vi "globals.vi"() -> ()   [LabVIEW 2011]
uses:
  relaySpec.ctl
  DA_Spec.ctl
  AD_Spec.ctl
panel:
  in  "Global Variables":enum32{"General", "Card Slots", "Functions"}(tab)=enum."Functions"
  out "GPIB Address":string="23"
  out "Log File Path":path
  out "Byte Stream File Refnum":refnum<file>
  out "Log String":string="00:00 Begin sequence\r\n00:01 R_H2:API_Iterations(\"1\"),API_Seq_Num(\"1/30\"),Active,Flow1(720),Remote\r\n00:01 H_Heater:API_Iterations(\"1\"),API_Repetitions(\"1\"),API_Seq_Num(\"2/30\"),Remote,Spinner\r\n00:06 A_Change_Temp_Setpoint:API_Description(\"100 C\"),API_ID(\"11\"),API_Iterations(\"1\"),API_Mode(\"Instantaneous\"),API_Seq_Num(\"3/30\"),API_Start,Elapsed Time \\(s\\)(\"0\"),Prompt(\"Is temperature 100 C?\"),Setpoint \\(C\\)(\"100\")\r\n00:08 H_Heater:API_Iterations(\"1\"),API_Repetitions(\"1\"),API_Seq_Num(\"4/30\"),Heater,Remote,Spinner\r\n00:38 A_Change_Temp_Setpoint:API_Description(\"200 C\"),API_ID(\"14\"),API_Iterations(\"1\"),API_Mode(\"Instantaneous\"),API_Seq_Num(\"5/30\"),API_Start,Elapsed Time \\(s\\)(\"0\"),Prompt(\"Is temperature 200 C?\"),Setpoint \\(C\\)(\"200\")\r\n01:38 A_Change_Temp_Setpoint:API_Description(\"300 C\"),API_ID(\"1\"),API_Iterations(\"1\"),API_Mode(\"Instantaneous\"),API_Seq_Num(\"6/30\"),API_Start,Elapsed Time \\(s\\)(\"0\"),Prompt(\"Is temperature 300 C?\"),Setpoint \\(C\\)(\"300\")\r\n01:39 A_III_V_Layer_v23:API_Calculated_Time(\"60\"),API_ID(\"12\"),API_Iterations(\"1\"),API_Mode(\"Finite\"),API_Seq_Num(\"7/30\"),API_Start,Al_bubbler.Flow(\"0\"),Al_bubbler.Name(\"Al\"),As_gas.Active,As_gas.Flow(\"8\"),As_gas.Name(\"As gas\"),Comment(\"fill lines\"),Ga_bubbler.Calculated(\"0\"),Ga_bubbler.MFC1 flow(\"10\"),Ga_bubbler.MFC2 flow(\"0\"),Ga_bubbler.MFC3 flow(\"0\"),Ga_bubbler.Main.Active,Ga_bubbler.Main.Flow(\"10\"),Ga_bubbler.Main.Name(\"Ga\"),In_bubbler.Active,In_bubbler.Flow(\"10\"),In_bubbler.Name(\"In\"),P_bubbler.Flow(\"0\"),P_bubbler.Name(\"P liq\"),P_gas.Active,P_gas.Flow(\"10\"),P_gas.Name(\"P gas\"),Se_bubbler.Calculated(\"0\"),Se_bubbler.MFC1 flow(\"0\"),Se_bubbler.MFC2 flow(\"10\"),Se_bubbler.MFC3 flow(\"100\"),Se_bubbler.Main.Flow(\"0\"),Se_bubbler.Main.Name(\"Se\"),Zn_bubbler.Calculated(\"0\"),Zn_bubbler.MFC1 flow(\"0\"),Zn_bubbler.MFC2 flow(\"10\"),Zn_bubbler.MFC3 flow(\"100\"),Zn_bubbler.Main.Flow(\"0\"),Zn_bubbler.Main.Name(\"Zn\"),prep_time(\"0\")\r\n02:39 A_III_V_Layer_v23:API_Calculated_Time(\"0\"),API_ID(\"6\"),API_Iterations(\"1\"),API_Mode(\"Finite\"),API_Seq_Num(\"8/30\"),API_Start,Al_bubbler.Flow(\"0\"),Al_bubbler.Name(\"Al\"),As_gas.Active,As_gas.Flow(\"4\"),As_gas.Name(\"As gas\"),As_gas.Prep,As_gas.Run,Comment(\"AsH3\"),Ga_bubbler.Calculated(\"0\"),Ga_bubbler.MFC1 flow(\"0\"),Ga_bubbler.MFC2 flow(\"0\"),Ga_bubbler.MFC3 flow(\"0\"),Ga_bubbler.Main.Flow(\"0\"),Ga_bubbler.Main.Name(\"Ga\"),In_bubbler.Flow(\"0\"),In_bubbler.Name(\"In\"),P_bubbler.Flow(\"0\"),P_bubbler.Name(\"P liq\"),P_gas.Flow(\"0\"),P_gas.Name(\"P gas\"),Se_bubbler.Calculated(\"0\"),Se_bubbler.MFC1 flow(\"0\"),Se_bubbler.MFC2 flow(\"10\"),Se_bubbler.MFC3 flow(\"100\"),Se_bubbler.Main.Flow(\"0\"),Se_bubbler.Main.Name(\"Se\"),Zn_bubbler.Calculated(\"0\"),Zn_bubbler.MFC1 flow(\"0\"),Zn_bubbler.MFC2 flow(\"10\"),Zn_bubbler.MFC3 flow(\"100\"),Zn_bubbler.Main.Flow(\"0\"),Zn_bubbler.Main.Name(\"Zn\"),prep_time(\"0\")\r\n02:39 A_Change_Temp_Setpoint:API_Description(\"400 C\"),API_ID(\"13\"),API_Iterations(\"1\"),API_Mode(\"Instantaneous\"),API_Seq_Num(\"9/30\"),API_Start,Elapsed Time \\(s\\)(\"0\"),Prompt(\"Is temperature 400 C?\"),Setpoint \\(C\\)(\"400\")\r\n03:39 A_Change_Temp_Setpoint:API_Description(\"500 C\"),API_ID(\"15\"),API_Iterations(\"1\"),API_Mode(\"Instantaneous\"),API_Seq_Num(\"10/30\"),API_Start,Elapsed Time \\(s\\)(\"0\"),Prompt(\"Is temperature 500 C?\"),Setpoint \\(C\\)(\"500\")\r\n04:40 A_Change_Temp_Setpoint:API_Description(\"600 C\"),API_ID(\"3\"),API_Iterations(\"1\"),API_Mode(\"Instantaneous\"),API_Seq_Num(\"11/30\"),API_Start,Elapsed Time \\(s\\)(\"0\"),Prompt(\"Is temperature 600 C?\"),Setpoint \\(C\\)(\"600\")\r\n05:40 A_Change_Temp_Setpoint:API_Description(\"625 C\"),API_ID(\"20\"),API_Iterations(\"1\"),API_Mode(\"Instantaneous\"),API_Seq_Num(\"12/30\"),API_Start,Elapsed Time \\(s\\)(\"0\"),Prompt(\"Is temperature 625 C?\"),Setpoint \\(C\\)(\"625\")\r\n06:40 A_III_V_Layer_v23:API_Calculated_Time(\"0\"),API_ID(\"2\"),API_Iterations(\"1\"),API_Mode(\"Finite\"),API_Seq_Num(\"13/30\"),API_Start,Al_bubbler.Flow(\"0\"),Al_bubbler.Name(\"Al\"),As_gas.Active,As_gas.Flow(\"4\"),As_gas.Name(\"As gas\"),As_gas.Prep,As_gas.Run,Comment(\"prep\"),Ga_bubbler.Calculated(\"0\"),Ga_bubbler.Dilution,Ga_bubbler.MFC1 flow(\"10\"),Ga_bubbler.MFC2 flow(\"10\"),Ga_bubbler.MFC3 flow(\"100\"),Ga_bubbler.Main.Active,Ga_bubbler.Main.Flow(\"0.909091\"),Ga_bubbler.Main.Name(\"Ga\"),In_bubbler.Flow(\"0\"),In_bubbler.Name(\"In\"),P_bubbler.Flow(\"0\"),P_bubbler.Name(\"P liq\"),P_gas.Flow(\"0\"),P_gas.Name(\"P gas\"),Se_bubbler.Calculated(\"0\"),Se_bubbler.MFC1 flow(\"0\"),Se_bubbler.MFC2 flow(\"10\"),Se_bubbler.MFC3 flow(\"100\"),Se_bubbler.Main.Flow(\"0\"),Se_bubbler.Main.Name(\"Se\"),Zn_bubbler.Calculated(\"0\"),Zn_bubbler.MFC1 flow(\"0\"),Zn_bubbler.MFC2 flow(\"10\"),Zn_bubbler.MFC3 flow(\"100\"),Zn_bubbler.Main.Flow(\"0\"),Zn_bubbler.Main.Name(\"Zn\"),prep_time(\"0\")\r\n06:40 A_Change_Temp_Setpoint:API_Description(\"650 C\"),API_ID(\"16\"),API_Iterations(\"1\"),API_Mode(\"Instantaneous\"),API_Seq_Num(\"14/30\"),API_Start,Elapsed Time \\(s\\)(\"0\"),Prompt(\"Is temperature 650 C?\"),Setpoint \\(C\\)(\"650\")\r\n07:40 A_III_V_Layer_v23:API_Calculated_Time(\"300\"),API_ID(\"21\"),API_Iterations(\"1\"),API_Mode(\"Finite\"),API_Seq_Num(\"15/30\"),API_Start,Al_bubbler.Flow(\"0\"),Al_bubbler.Name(\"Al\"),As_gas.Active,As_gas.Flow(\"6\"),As_gas.Name(\"As gas\"),As_gas.Prep,As_gas.Run,Comment(\"GaAs buffer 1\"),Ga_bubbler.Calculated(\"0\"),Ga_bubbler.Dilution,Ga_bubbler.MFC1 flow(\"10\"),Ga_bubbler.MFC2 flow(\"10\"),Ga_bubbler.MFC3 flow(\"100\"),Ga_bubbler.Main.Active,Ga_bubbler.Main.Flow(\"0.909091\"),Ga_bubbler.Main.Name(\"Ga\"),Ga_bubbler.Main.Run,In_bubbler.Flow(\"0\"),In_bubbler.Name(\"In\"),P_bubbler.Flow(\"0\"),P_bubbler.Name(\"P liq\"),P_gas.Flow(\"0\"),P_gas.Name(\"P gas\"),Se_bubbler.Calculated(\"0\"),Se_bubbler.MFC1 flow(\"0\"),Se_bubbler.MFC2 flow(\"10\"),Se_bubbler.MFC3 flow(\"100\"),Se_bubbler.Main.Flow(\"0\"),Se_bubbler.Main.Name(\"Se\"),Zn_bubbler.Calculated(\"0\"),Zn_bubbler.MFC1 flow(\"0\"),Zn_bubbler.MFC2 flow(\"10\"),Zn_bubbler.MFC3 flow(\"100\"),Zn_bubbler.Main.Flow(\"0\"),Zn_bubbler.Main.Name(\"Zn\"),prep_time(\"60\")\r\n12:41 A_III_V_Layer_v23:API_Calculated_Time(\"124\"),API_ID(\"18\"),API_Iterations(\"1\"),API_Mode(\"Finite\"),API_Seq_Num(\"16/30\"),API_Start,Al_bubbler.Flow(\"0\"),Al_bubbler.Name(\"Al\"),As_gas.Active,As_gas.Flow(\"6\"),As_gas.Name(\"As gas\"),As_gas.Prep,As_gas.Run,Comment(\"GaAs buffer2\"),Ga_bubbler.Calculated(\"0\"),Ga_bubbler.Dilution,Ga_bubbler.MFC1 flow(\"10\"),Ga_bubbler.MFC2 flow(\"10\"),Ga_bubbler.MFC3 flow(\"100\"),Ga_bubbler.Main.Active,Ga_bubbler.Main.Flow(\"0.909091\"),Ga_bubbler.Main.Name(\"Ga\"),Ga_bubbler.Main.Run,In_bubbler.Active,In_bubbler.Flow(\"70\"),In_bubbler.Name(\"In\"),P_bubbler.Flow(\"0\"),P_bubbler.Name(\"P liq\"),P_gas.Active,P_gas.Flow(\"4\"),P_gas.Name(\"P gas\"),Se_bubbler.Calculated(\"0\"),Se_bubbler.MFC1 flow(\"0\"),Se_bubbler.MFC2 flow(\"10\"),Se_bubbler.MFC3 flow(\"100\"),Se_bubbler.Main.Flow(\"0\"),Se_bubbler.Main.Name(\"Se\"),Zn_bubbler.Calculated(\"0\"),Zn_bubbler.MFC1 flow(\"0\"),Zn_bubbler.MFC2 flow(\"10\"),Zn_bubbler.MFC3 flow(\"100\"),Zn_bubbler.Main.Flow(\"0\"),Zn_bubbler.Main.Name(\"Zn\"),prep_time(\"4\")\r\n14:46 A_III_V_Layer_v23:API_Calculated_Time(\"2\"),API_ID(\"8\"),API_Iterations(\"1\"),API_Mode(\"Finite\"),API_Seq_Num(\"17/30\"),API_Start,Al_bubbler.Flow(\"0\"),Al_bubbler.Name(\"Al\"),As_gas.Active,As_gas.Flow(\"4\"),As_gas.Name(\"As gas\"),As_gas.Prep,As_gas.Run,Comment(\"post buffer 2\"),Ga_bubbler.Calculated(\"0\"),Ga_bubbler.Dilution,Ga_bubbler.MFC1 flow(\"9.56\"),Ga_bubbler.MFC2 flow(\"10\"),Ga_bubbler.MFC3 flow(\"100\"),Ga_bubbler.Main.Active,Ga_bubbler.Main.Flow(\"0.872581\"),Ga_bubbler.Main.Name(\"Ga\"),In_bubbler.Active,In_bubbler.Flow(\"70\"),In_bubbler.Name(\"In\"),P_bubbler.Flow(\"0\"),P_bubbler.Name(\"P liq\"),P_gas.Active,P_gas.Flow(\"4\"),P_gas.Name(\"P gas\"),Se_bubbler.Calculated(\"0\"),Se_bubbler.MFC1 flow(\"0\"),Se_bubbler.MFC2 flow(\"10\"),Se_bubbler.MFC3 flow(\"100\"),Se_bubbler.Main.Flow(\"0\"),Se_bubbler.Main.Name(\"Se\"),Zn_bubbler.Calculated(\"0\"),Zn_bubbler.MFC1 flow(\"0\"),Zn_bubbler.MFC2 flow(\"10\"),Zn_bubbler.MFC3 flow(\"100\"),Zn_bubbler.Main.Flow(\"0\"),Zn_bubbler.Main.Name(\"Zn\"),prep_time(\"0\")\r\n14:48 A_III_V_Layer_v23:API_Calculated_Time(\"2\"),API_ID(\"9\"),API_Iterations(\"1\"),API_Mode(\"Finite\"),API_Seq_Num(\"18/30\"),API_Start,Al_bubbler.Flow(\"0\"),Al_bubbler.Name(\"Al\"),As_gas.Flow(\"0\"),As_gas.Name(\"As gas\"),Comment(\"nothing running\"),Ga_bubbler.Calculated(\"0\"),Ga_bubbler.Dilution,Ga_bubbler.MFC1 flow(\"9.56\"),Ga_bubbler.MFC2 flow(\"10\"),Ga_bubbler.MFC3 flow(\"100\"),Ga_bubbler.Main.Active,Ga_bubbler.Main.Flow(\"0.872581\"),Ga_bubbler.Main.Name(\"Ga\"),In_bubbler.Active,In_bubbler.Flow(\"70\"),In_bubbler.Name(\"In\"),P_bubbler.Flow(\"0\"),P_bubbler.Name(\"P liq\"),P_gas.Active,P_gas.Flow(\"4\"),P_gas.Name(\"P gas\"),Se_bubbler.Calculated(\"0\"),Se_bubbler.MFC1 flow(\"0\"),Se_bubbler.MFC2 flow(\"10\"),Se_bubbler.MFC3 flow(\"100\"),Se_bubbler.Main.Flow(\"0\"),Se_bubbler.Main.Name(\"Se\"),Zn_bubbler.Calculated(\"0\"),Zn_bubbler.MFC1 flow(\"0\"),Zn_bubbler.MFC2 flow(\"10\"),Zn_bubbler.MFC3 flow(\"100\"),Zn_bubbler.Main.Flow(\"0\"),Zn_bubbler.Main.Name(\"Zn\"),prep_time(\"0\")\r\n14:50 A_III_V_Layer_v23:API_Calculated_Time(\"3484\"),API_ID(\"19\"),API_Iterations(\"1\"),API_Mode(\"Finite\"),API_Seq_Num(\"19/30\"),API_Start,Al_bubbler.Flow(\"0\"),Al_bubbler.Name(\"Al\"),As_gas.Flow(\"0\"),As_gas.Name(\"As gas\"),Comment(\"GaInP\"),Ga_bubbler.Calculated(\"0\"),Ga_bubbler.Dilution,Ga_bubbler.MFC1 flow(\"9.56\"),Ga_bubbler.MFC2 flow(\"10\"),Ga_bubbler.MFC3 flow(\"100\"),Ga_bubbler.Main.Active,Ga_bubbler.Main.Flow(\"0.872581\"),Ga_bubbler.Main.Name(\"Ga\"),Ga_bubbler.Main.Run,In_bubbler.Active,In_bubbler.Flow(\"70\"),In_bubbler.Name(\"In\"),In_bubbler.Run,P_bubbler.Flow(\"0\"),P_bubbler.Name(\"P liq\"),P_gas.Active,P_gas.Flow(\"4\"),P_gas.Name(\"P gas\"),P_gas.Prep,P_gas.Run,Se_bubbler.Calculated(\"0\"),Se_bubbler.MFC1 flow(\"0\"),Se_bubbler.MFC2 flow(\"10\"),Se_bubbler.MFC3 flow(\"100\"),Se_bubbler.Main.Flow(\"0\"),Se_bubbler.Main.Name(\"Se\"),Zn_bubbler.Calculated(\"0\"),Zn_bubbler.MFC1 flow(\"0\"),Zn_bubbler.MFC2 flow(\"10\"),Zn_bubbler.MFC3 flow(\"100\"),Zn_bubbler.Main.Flow(\"0\"),Zn_bubbler.Main.Name(\"Zn\"),prep_time(\"4\")\r\n1:22:42 A_III_V_Layer_v23:API_Calculated_Time(\"120\"),API_ID(\"22\"),API_Iterations(\"1\"),API_Mode(\"Finite\"),API_Seq_Num(\"20/30\"),API_Start,Al_bubbler.Flow(\"0\"),Al_bubbler.Name(\"Al\"),As_gas.Active,As_gas.Flow(\"4\"),As_gas.Name(\"As gas\"),Comment(\"GaInP_end\"),Ga_bubbler.Calculated(\"0\"),Ga_bubbler.Dilution,Ga_bubbler.MFC1 flow(\"9.56\"),Ga_bubbler.MFC2 flow(\"10\"),Ga_bubbler.MFC3 flow(\"100\"),Ga_bubbler.Main.Active,Ga_bubbler.Main.Flow(\"0.872581\"),Ga_bubbler.Main.Name(\"Ga\"),Ga_bubbler.Main.Run,In_bubbler.Active,In_bubbler.Flow(\"70\"),In_bubbler.Name(\"In\"),In_bubbler.Run,P_bubbler.Flow(\"0\"),P_bubbler.Name(\"P liq\"),P_gas.Active,P_gas.Flow(\"4\"),P_gas.Name(\"P gas\"),P_gas.Prep,P_gas.Run,Se_bubbler.Calculated(\"0\"),Se_bubbler.MFC1 flow(\"0\"),Se_bubbler.MFC2 flow(\"10\"),Se_bubbler.MFC3 flow(\"100\"),Se_bubbler.Main.Flow(\"0\"),Se_bubbler.Main.Name(\"Se\"),Zn_bubbler.Calculated(\"0\"),Zn_bubbler.MFC1 flow(\"0\"),Zn_bubbler.MFC2 flow(\"10\"),Zn_bubbler.MFC3 flow(\"100\"),Zn_bubbler.Main.Flow(\"0\"),Zn_bubbler.Main.Name(\"Zn\"),prep_time(\"0\")\r\n1:24:42 A_III_V_Layer_v23:API_Calculated_Time(\"4\"),API_ID(\"23\"),API_Iterations(\"1\"),API_Mode(\"Finite\"),API_Seq_Num(\"21/30\"),API_Start,Al_bubbler.Flow(\"0\"),Al_bubbler.Name(\"Al\"),As_gas.Active,As_gas.Flow(\"4\"),As_gas.Name(\"As gas\"),Comment(\"post-GaInP\"),Ga_bubbler.Calculated(\"0\"),Ga_bubbler.Dilution,Ga_bubbler.MFC1 flow(\"10\"),Ga_bubbler.MFC2 flow(\"10\"),Ga_bubbler.MFC3 flow(\"100\"),Ga_bubbler.Main.Active,Ga_bubbler.Main.Flow(\"0.909091\"),Ga_bubbler.Main.Name(\"Ga\"),In_bubbler.Flow(\"0\"),In_bubbler.Name(\"In\"),P_bubbler.Flow(\"0\"),P_bubbler.Name(\"P liq\"),P_gas.Active,P_gas.Flow(\"4\"),P_gas.Name(\"P gas\"),P_gas.Prep,P_gas.Run,Se_bubbler.Calculated(\"0\"),Se_bubbler.MFC1 flow(\"0\"),Se_bubbler.MFC2 flow(\"10\"),Se_bubbler.MFC3 flow(\"100\"),Se_bubbler.Main.Flow(\"0\"),Se_bubbler.Main.Name(\"Se\"),Zn_bubbler.Calculated(\"0\"),Zn_bubbler.MFC1 flow(\"0\"),Zn_bubbler.MFC2 flow(\"10\"),Zn_bubbler.MFC3 flow(\"100\"),Zn_bubbler.Main.Flow(\"0\"),Zn_bubbler.Main.Name(\"Zn\"),prep_time(\"0\")\r\n1:24:46 A_III_V_Layer_v23:API_Calculated_Time(\"2\"),API_ID(\"4\"),API_Iterations(\"1\"),API_Mode(\"Finite\"),API_Seq_Num(\"22/30\"),API_Start,Al_bubbler.Flow(\"0\"),Al_bubbler.Name(\"Al\"),As_gas.Active,As_gas.Flow(\"4\"),As_gas.Name(\"As gas\"),Comment(\"no growth\"),Ga_bubbler.Calculated(\"0\"),Ga_bubbler.Dilution,Ga_bubbler.MFC1 flow(\"10\"),Ga_bubbler.MFC2 flow(\"10\"),Ga_bubbler.MFC3 flow(\"100\"),Ga_bubbler.Main.Active,Ga_bubbler.Main.Flow(\"0.909091\"),Ga_bubbler.Main.Name(\"Ga\"),In_bubbler.Flow(\"0\"),In_bubbler.Name(\"In\"),P_bubbler.Flow(\"0\"),P_bubbler.Name(\"P liq\"),P_gas.Flow(\"0\"),P_gas.Name(\"P gas\"),Se_bubbler.Calculated(\"0\"),Se_bubbler.MFC1 flow(\"0\"),Se_bubbler.MFC2 flow(\"10\"),Se_bubbler.MFC3 flow(\"100\"),Se_bubbler.Main.Flow(\"0\"),Se_bubbler.Main.Name(\"Se\"),Zn_bubbler.Calculated(\"0\"),Zn_bubbler.MFC1 flow(\"0\"),Zn_bubbler.MFC2 flow(\"10\"),Zn_bubbler.MFC3 flow(\"100\"),Zn_bubbler.Main.Flow(\"0\"),Zn_bubbler.Main.Name(\"Zn\"),prep_time(\"2\")\r\n1:24:49 A_III_V_Layer_v23:API_Calculated_Time(\"125\"),API_ID(\"5\"),API_Iterations(\"1\"),API_Mode(\"Finite\"),API_Seq_Num(\"23/30\"),API_Start,Al_bubbler.Flow(\"0\"),Al_bubbler.Name(\"Al\"),As_gas.Active,As_gas.Flow(\"4\"),As_gas.Name(\"As gas\"),As_gas.Prep,As_gas.Run,Comment(\"cap\"),Ga_bubbler.Calculated(\"0\"),Ga_bubbler.Dilution,Ga_bubbler.MFC1 flow(\"10\"),Ga_bubbler.MFC2 flow(\"10\"),Ga_bubbler.MFC3 flow(\"100\"),Ga_bubbler.Main.Active,Ga_bubbler.Main.Flow(\"0.909091\"),Ga_bubbler.Main.Name(\"Ga\"),Ga_bubbler.Main.Run,In_bubbler.Flow(\"0\"),In_bubbler.Name(\"In\"),P_bubbler.Flow(\"0\"),P_bubbler.Name(\"P liq\"),P_gas.Flow(\"0\"),P_gas.Name(\"P gas\"),Se_bubbler.Calculated(\"0\"),Se_bubbler.MFC1 flow(\"0\"),Se_bubbler.MFC2 flow(\"10\"),Se_bubbler.MFC3 flow(\"100\"),Se_bubbler.Main.Flow(\"0\"),Se_bubbler.Main.Name(\"Se\"),Zn_bubbler.Calculated(\"0\"),Zn_bubbler.MFC1 flow(\"0\"),Zn_bubbler.MFC2 flow(\"10\"),Zn_bubbler.MFC3 flow(\"100\"),Zn_bubbler.Main.Flow(\"0\"),Zn_bubbler.Main.Name(\"Zn\"),prep_time(\"5\")\r\n1:26:55 A_III_V_Layer_v23:API_Calculated_Time(\"0\"),API_ID(\"10\"),API_Iterations(\"1\"),API_Mode(\"Finite\"),API_Seq_Num(\"24/30\"),API_Start,Al_bubbler.Flow(\"0\"),Al_bubbler.Name(\"Al\"),As_gas.Active,As_gas.Flow(\"3\"),As_gas.Name(\"As gas\"),As_gas.Prep,As_gas.Run,Comment(\"post growth\"),Ga_bubbler.Calculated(\"0\"),Ga_bubbler.MFC1 flow(\"0\"),Ga_bubbler.MFC2 flow(\"0\"),Ga_bubbler.MFC3 flow(\"0\"),Ga_bubbler.Main.Flow(\"0\"),Ga_bubbler.Main.Name(\"Ga\"),In_bubbler.Flow(\"0\"),In_bubbler.Name(\"In\"),P_bubbler.Flow(\"0\"),P_bubbler.Name(\"P liq\"),P_gas.Flow(\"0\"),P_gas.Name(\"P gas\"),Se_bubbler.Calculated(\"0\"),Se_bubbler.MFC1 flow(\"0\"),Se_bubbler.MFC2 flow(\"10\"),Se_bubbler.MFC3 flow(\"100\"),Se_bubbler.Main.Flow(\"0\"),Se_bubbler.Main.Name(\"Se\"),Zn_bubbler.Calculated(\"0\"),Zn_bubbler.MFC1 flow(\"0\"),Zn_bubbler.MFC2 flow(\"10\"),Zn_bubbler.MFC3 flow(\"100\"),Zn_bubbler.Main.Flow(\"0\"),Zn_bubbler.Main.Name(\"Zn\"),prep_time(\"0\")\r\n1:26:55 A_Change_Temp_Setpoint:API_Description(\"20 C\"),API_ID(\"7\"),API_Iterations(\"1\"),API_Mode(\"Instantaneous\"),API_Seq_Num(\"25/30\"),API_Start,Elapsed Time \\(s\\)(\"0\"),Prompt(\"Is temperature 20 C?\"),Setpoint \\(C\\)(\"20\")\r\n1:26:55 H_Heater:API_Iterations(\"1\"),API_Repetitions(\"1\"),API_Seq_Num(\"26/30\"),Comment(\"Heater Off\"),Remote,Spinner\r\n1:31:55 A_FlushAndShutOff_v02:API_Calculated_Time(\"120\"),API_Description(\"Default\"),API_ID(\"17\"),API_Iterations(\"1\"),API_Mode(\"Finite\"),API_Seq_Num(\"27/30\"),API_Start,Al Flow(\"0\"),AsH3 Flow(\"10\"),Ga Flow(\"10\"),In Flow(\"20\"),P Flow(\"20\"),P Liq Flow(\"0\"),Se Flow(\"0\"),Zn Flow(\"0\"),is OK?,tTotal\\(s\\) 2(\"0\"),total time(\"0\")\r\n1:33:26 R_H2:API_Iterations(\"1\"),API_Repetitions(\"1\"),API_Seq_Num(\"28/30\"),Active,Comment(\"reduce H2\\, continue cool down\"),Flow1(360),Remote\r\n1:38:30 H_Heater:API_Iterations(\"1\"),API_Repetitions(\"1\"),API_Seq_Num(\"29/30\")\r\n1:38:31 R_H2:API_Iterations(\"1\"),API_Repetitions(\"1\"),API_Seq_Num(\"30/30\")\r\n1:38:31 End Sequence\r\n"
  out "Temperature Controller RS232":refnum<visa-resource-name>="COM1"
  out "Begin Time":timestamp=timestamp(3704976602.8778777 s since 1904-01-01)
  out "Current Time":timestamp=timestamp(3704982512.995525 s since 1904-01-01)
  out "Seq Step Time (s)":dbl=0.1
  out "Last Step":i32=29
  out "Log Path":path=path "C:/MOCVD/Log Files/210527a_GaInP.txt"
  out "Growth Database":path=path "C:/MOCVD/MOCVD_Growths.accdb"
  out "Growth Sequence Preferences":path=path "C:/MOCVD/GrowthSequencePreferences.ini"
  in  "Multiprogrammer Card Slots":T1={"Relay Card Slots"={"Card 1"=10, "Card 2"=11, "Card 3"=12, "Card 4"=13, "Card 5"=14}, "A/D Card Slots"={"Scanner"=0, "High-Speed A/D"=1, "Timer"=2}, "D/A Cards"={"Quad (10-bit) D/A Card Slots"={"Card 1"=4, "Card 2"=5, "Card 3"=7, "Card 4"=8, "Card 5"=9}, "Single (12-bit) D/A Card Slot"={"Card 6"=6}}} {"D/A Cards"."Single (12-bit) D/A Card Slot"."Card 6" items=["400@", "401A", "402B", "403C", "404D", "405E", "406F", "407G", "408H", "409I", "410J", "411K", "412L", "413M", "414N"]; "D/A Cards"."Quad (10-bit) D/A Card Slots"."Card 1" items=["400@", "401A", "402B", "403C", "404D", "405E", "406F", "407G", "408H", "409I", "410J", "411K", "412L", "413M", "414N"]; "D/A Cards"."Quad (10-bit) D/A Card Slots"."Card 2" items=["400@", "401A", "402B", "403C", "404D", "405E", "406F", "407G", "408H", "409I", "410J", "411K", "412L", "413M", "414N"]; "D/A Cards"."Quad (10-bit) D/A Card Slots"."Card 3" items=["400@", "401A", "402B", "403C", "404D", "405E", "406F", "407G", "408H", "409I", "410J", "411K", "412L", "413M", "414N"]; "D/A Cards"."Quad (10-bit) D/A Card Slots"."Card 4" items=["400@", "401A", "402B", "403C", "404D", "405E", "406F", "407G", "408H", "409I", "410J", "411K", "412L", "413M", "414N"]; "D/A Cards"."Quad (10-bit) D/A Card Slots"."Card 5" items=["400@", "401A", "402B", "403C", "404D", "405E", "406F", "407G", "408H", "409I", "410J", "411K", "412L", "413M", "414N"]; "A/D Card Slots"."Timer" items=["400@", "401A", "402B", "403C", "404D", "405E", "406F", "407G", "408H", "409I", "410J", "411K", "412L", "413M", "414N"]; "A/D Card Slots"."High-Speed A/D" items=["400@", "401A", "402B", "403C", "404D", "405E", "406F", "407G", "408H", "409I", "410J", "411K", "412L", "413M", "414N"]; "A/D Card Slots"."Scanner" items=["400@", "401A", "402B", "403C", "404D", "405E", "406F", "407G", "408H", "409I", "410J", "411K", "412L", "413M", "414N"]; "Relay Card Slots"."Card 5" items=["400@", "401A", "402B", "403C", "404D", "405E", "406F", "407G", "408H", "409I", "410J", "411K", "412L", "413M", "414N"]; "Relay Card Slots"."Card 4" items=["400@", "401A", "402B", "403C", "404D", "405E", "406F", "407G", "408H", "409I", "410J", "411K", "412L", "413M", "414N"]; "Relay Card Slots"."Card 3" items=["400@", "401A", "402B", "403C", "404D", "405E", "406F", "407G", "408H", "409I", "410J", "411K", "412L", "413M", "414N"]; "Relay Card Slots"."Card 2" items=["400@", "401A", "402B", "403C", "404D", "405E", "406F", "407G", "408H", "409I", "410J", "411K", "412L", "413M", "414N"]; "Relay Card Slots"."Card 1" items=["400@", "401A", "402B", "403C", "404D", "405E", "406F", "407G", "408H", "409I", "410J", "411K", "412L", "413M", "414N"]}
  in  "Functions":T2(tab)=enum."As gas"
  in  "H2/N2":T6={"Relay Functions"={"Remote"={"Card Index"=0, "Relay Index"=0}, "H2 active"={"Card Index"=0, "Relay Index"=1}, "N2 active"={"Card Index"=0, "Relay Index"=2}, "Output"={"Card Index"=0, "Relay Index"=11}}, "D/A Functions"={"H2 flow"={"Card Index"=0, "Channel Index"=1}, "N2 flow"={"Card Index"=0, "Channel Index"=0}}, "Flow Ranges"={"H2 flow (HMFC1)"=2, "N2 flow (NMFC1)"=2}, "A/D Functions"={"H2/N2 flow"=0}} {"A/D Functions"."H2/N2 flow" items=["Channel 1", "Channel 2", "Channel 3", "Channel 4", "Channel 5", "Channel 6", "Channel 7", "Channel 8", "Channel 9", "Channel 10", "Channel 11", "Channel 12", "Channel 13", "Channel 14", "Channel 15", "Channel 16"]; "Flow Ranges"."N2 flow (NMFC1)" items=["0-10 sccm", "0-100 sccm", "0-1000 sccm"]; "Flow Ranges"."H2 flow (HMFC1)" items=["0-10 sccm", "0-100 sccm", "0-1000 sccm"]; "D/A Functions"."N2 flow"."Card Index" items=["Card 1", "Card 2", "Card 3", "Card 4", "Card 5", "Card 6"]; "D/A Functions"."N2 flow"."Channel Index" items=["Channel 1", "Channel 2", "Channel 3", "Channel 4"]; "D/A Functions"."H2 flow"."Card Index" items=["Card 1", "Card 2", "Card 3", "Card 4", "Card 5", "Card 6"]; "D/A Functions"."H2 flow"."Channel Index" items=["Channel 1", "Channel 2", "Channel 3", "Channel 4"]; "Relay Functions"."Output"."Card Index" items=["Card 1", "Card 2", "Card 3", "Card 4", "Card 5"]; "Relay Functions"."Output"."Relay Index" items=["Relay 1", "Relay 2", "Relay 3", "Relay 4", "Relay 5", "Relay 6", "Relay 7", "Relay 8", "Relay 9", "Relay 10", "Relay 11", "Relay 12"]; "Relay Functions"."N2 active"."Card Index" items=["Card 1", "Card 2", "Card 3", "Card 4", "Card 5"]; "Relay Functions"."N2 active"."Relay Index" items=["Relay 1", "Relay 2", "Relay 3", "Relay 4", "Relay 5", "Relay 6", "Relay 7", "Relay 8", "Relay 9", "Relay 10", "Relay 11", "Relay 12"]; "Relay Functions"."H2 active"."Card Index" items=["Card 1", "Card 2", "Card 3", "Card 4", "Card 5"]; "Relay Functions"."H2 active"."Relay Index" items=["Relay 1", "Relay 2", "Relay 3", "Relay 4", "Relay 5", "Relay 6", "Relay 7", "Relay 8", "Relay 9", "Relay 10", "Relay 11", "Relay 12"]; "Relay Functions"."Remote"."Card Index" items=["Card 1", "Card 2", "Card 3", "Card 4", "Card 5"]; "Relay Functions"."Remote"."Relay Index" items=["Relay 1", "Relay 2", "Relay 3", "Relay 4", "Relay 5", "Relay 6", "Relay 7", "Relay 8", "Relay 9", "Relay 10", "Relay 11", "Relay 12"]}
  in  "Al":T7={"Relay Functions"={"Remote"={"Card Index"=0, "Relay Index"=3}, "Active"={"Card Index"=0, "Relay Index"=4}, "Bubbler In"={"Card Index"=0, "Relay Index"=5}, "Run"={"Card Index"=0, "Relay Index"=6}}, "D/A Functions"={"Flow"={"Card Index"=3, "Channel Index"=0}}, "Flow Ranges"={"Flow (AlMFC1)"=1}, "A/D Functions"={"Flow"=1}} {"A/D Functions"."Flow" items=["Channel 1", "Channel 2", "Channel 3", "Channel 4", "Channel 5", "Channel 6", "Channel 7", "Channel 8", "Channel 9", "Channel 10", "Channel 11", "Channel 12", "Channel 13", "Channel 14", "Channel 15", "Channel 16"]; "Flow Ranges"."Flow (AlMFC1)" items=["0-10 sccm", "0-100 sccm", "0-1000 sccm"]; "D/A Functions"."Flow"."Card Index" items=["Card 1", "Card 2", "Card 3", "Card 4", "Card 5", "Card 6"]; "D/A Functions"."Flow"."Channel Index" items=["Channel 1", "Channel 2", "Channel 3", "Channel 4"]; "Relay Functions"."Run"."Card Index" items=["Card 1", "Card 2", "Card 3", "Card 4", "Card 5"]; "Relay Functions"."Run"."Relay Index" items=["Relay 1", "Relay 2", "Relay 3", "Relay 4", "Relay 5", "Relay 6", "Relay 7", "Relay 8", "Relay 9", "Relay 10", "Relay 11", "Relay 12"]; "Relay Functions"."Bubbler In"."Card Index" items=["Card 1", "Card 2", "Card 3", "Card 4", "Card 5"]; "Relay Functions"."Bubbler In"."Relay Index" items=["Relay 1", "Relay 2", "Relay 3", "Relay 4", "Relay 5", "Relay 6", "Relay 7", "Relay 8", "Relay 9", "Relay 10", "Relay 11", "Relay 12"]; "Relay Functions"."Active"."Card Index" items=["Card 1", "Card 2", "Card 3", "Card 4", "Card 5"]; "Relay Functions"."Active"."Relay Index" items=["Relay 1", "Relay 2", "Relay 3", "Relay 4", "Relay 5", "Relay 6", "Relay 7", "Relay 8", "Relay 9", "Relay 10", "Relay 11", "Relay 12"]; "Relay Functions"."Remote"."Card Index" items=["Card 1", "Card 2", "Card 3", "Card 4", "Card 5"]; "Relay Functions"."Remote"."Relay Index" items=["Relay 1", "Relay 2", "Relay 3", "Relay 4", "Relay 5", "Relay 6", "Relay 7", "Relay 8", "Relay 9", "Relay 10", "Relay 11", "Relay 12"]}
  in  "Ga":T8={"Relay Functions"={"Remote"={"Card Index"=3, "Relay Index"=0}, "Active"={"Card Index"=3, "Relay Index"=1}, "Bubbler In"={"Card Index"=3, "Relay Index"=2}, "H2 dilute"={"Card Index"=3, "Relay Index"=4}, "Run"={"Card Index"=3, "Relay Index"=3}}, "D/A Functions"={"Flow 1"={"Card Index"=4, "Channel Index"=0}, "Flow 2"={"Card Index"=4, "Channel Index"=1}, "Flow 3"={"Card Index"=4, "Channel Index"=2}}, "Flow Ranges"={"Flow 1 (GAMFC1)"=0, "Flow 2 (GAMFC2)"=1, "Flow 3 (GAMFC3)"=2}, "A/D Functions"={"Flow 1"=3, "Flow 2"=4, "Flow 3"=7}} {"A/D Functions"."Flow 3" items=["Channel 1", "Channel 2", "Channel 3", "Channel 4", "Channel 5", "Channel 6", "Channel 7", "Channel 8", "Channel 9", "Channel 10", "Channel 11", "Channel 12", "Channel 13", "Channel 14", "Channel 15", "Channel 16"]; "A/D Functions"."Flow 2" items=["Channel 1", "Channel 2", "Channel 3", "Channel 4", "Channel 5", "Channel 6", "Channel 7", "Channel 8", "Channel 9", "Channel 10", "Channel 11", "Channel 12", "Channel 13", "Channel 14", "Channel 15", "Channel 16"]; "A/D Functions"."Flow 1" items=["Channel 1", "Channel 2", "Channel 3", "Channel 4", "Channel 5", "Channel 6", "Channel 7", "Channel 8", "Channel 9", "Channel 10", "Channel 11", "Channel 12", "Channel 13", "Channel 14", "Channel 15", "Channel 16"]; "Flow Ranges"."Flow 3 (GAMFC3)" items=["0-10 sccm", "0-100 sccm", "0-1000 sccm"]; "Flow Ranges"."Flow 2 (GAMFC2)" items=["0-10 sccm", "0-100 sccm", "0-1000 sccm"]; "Flow Ranges"."Flow 1 (GAMFC1)" items=["0-10 sccm", "0-100 sccm", "0-1000 sccm"]; "D/A Functions"."Flow 3"."Card Index" items=["Card 1", "Card 2", "Card 3", "Card 4", "Card 5", "Card 6"]; "D/A Functions"."Flow 3"."Channel Index" items=["Channel 1", "Channel 2", "Channel 3", "Channel 4"]; "D/A Functions"."Flow 2"."Card Index" items=["Card 1", "Card 2", "Card 3", "Card 4", "Card 5", "Card 6"]; "D/A Functions"."Flow 2"."Channel Index" items=["Channel 1", "Channel 2", "Channel 3", "Channel 4"]; "D/A Functions"."Flow 1"."Card Index" items=["Card 1", "Card 2", "Card 3", "Card 4", "Card 5", "Card 6"]; "D/A Functions"."Flow 1"."Channel Index" items=["Channel 1", "Channel 2", "Channel 3", "Channel 4"]; "Relay Functions"."Run"."Card Index" items=["Card 1", "Card 2", "Card 3", "Card 4", "Card 5"]; "Relay Functions"."Run"."Relay Index" items=["Relay 1", "Relay 2", "Relay 3", "Relay 4", "Relay 5", "Relay 6", "Relay 7", "Relay 8", "Relay 9", "Relay 10", "Relay 11", "Relay 12"]; "Relay Functions"."H2 dilute"."Card Index" items=["Card 1", "Card 2", "Card 3", "Card 4", "Card 5"]; "Relay Functions"."H2 dilute"."Relay Index" items=["Relay 1", "Relay 2", "Relay 3", "Relay 4", "Relay 5", "Relay 6", "Relay 7", "Relay 8", "Relay 9", "Relay 10", "Relay 11", "Relay 12"]; "Relay Functions"."Bubbler In"."Card Index" items=["Card 1", "Card 2", "Card 3", "Card 4", "Card 5"]; "Relay Functions"."Bubbler In"."Relay Index" items=["Relay 1", "Relay 2", "Relay 3", "Relay 4", "Relay 5", "Relay 6", "Relay 7", "Relay 8", "Relay 9", "Relay 10", "Relay 11", "Relay 12"]; "Relay Functions"."Active"."Card Index" items=["Card 1", "Card 2", "Card 3", "Card 4", "Card 5"]; "Relay Functions"."Active"."Relay Index" items=["Relay 1", "Relay 2", "Relay 3", "Relay 4", "Relay 5", "Relay 6", "Relay 7", "Relay 8", "Relay 9", "Relay 10", "Relay 11", "Relay 12"]; "Relay Functions"."Remote"."Card Index" items=["Card 1", "Card 2", "Card 3", "Card 4", "Card 5"]; "Relay Functions"."Remote"."Relay Index" items=["Relay 1", "Relay 2", "Relay 3", "Relay 4", "Relay 5", "Relay 6", "Relay 7", "Relay 8", "Relay 9", "Relay 10", "Relay 11", "Relay 12"]}
  in  "In":T9={"Relay Functions"={"Remote"={"Card Index"=0, "Relay Index"=7}, "Active"={"Card Index"=0, "Relay Index"=8}, "Bubbler In"={"Card Index"=0, "Relay Index"=9}, "Run"={"Card Index"=0, "Relay Index"=10}}, "D/A Functions"={"Flow"={"Card Index"=0, "Channel Index"=3}}, "Flow Ranges"={"Flow (INMFC1)"=1}, "A/D Functions"={"Flow"=2}} {"A/D Functions"."Flow" items=["Channel 1", "Channel 2", "Channel 3", "Channel 4", "Channel 5", "Channel 6", "Channel 7", "Channel 8", "Channel 9", "Channel 10", "Channel 11", "Channel 12", "Channel 13", "Channel 14", "Channel 15", "Channel 16"]; "Flow Ranges"."Flow (INMFC1)" items=["0-10 sccm", "0-100 sccm", "0-1000 sccm"]; "D/A Functions"."Flow"."Card Index" items=["Card 1", "Card 2", "Card 3", "Card 4", "Card 5", "Card 6"]; "D/A Functions"."Flow"."Channel Index" items=["Channel 1", "Channel 2", "Channel 3", "Channel 4"]; "Relay Functions"."Run"."Card Index" items=["Card 1", "Card 2", "Card 3", "Card 4", "Card 5"]; "Relay Functions"."Run"."Relay Index" items=["Relay 1", "Relay 2", "Relay 3", "Relay 4", "Relay 5", "Relay 6", "Relay 7", "Relay 8", "Relay 9", "Relay 10", "Relay 11", "Relay 12"]; "Relay Functions"."Bubbler In"."Card Index" items=["Card 1", "Card 2", "Card 3", "Card 4", "Card 5"]; "Relay Functions"."Bubbler In"."Relay Index" items=["Relay 1", "Relay 2", "Relay 3", "Relay 4", "Relay 5", "Relay 6", "Relay 7", "Relay 8", "Relay 9", "Relay 10", "Relay 11", "Relay 12"]; "Relay Functions"."Active"."Card Index" items=["Card 1", "Card 2", "Card 3", "Card 4", "Card 5"]; "Relay Functions"."Active"."Relay Index" items=["Relay 1", "Relay 2", "Relay 3", "Relay 4", "Relay 5", "Relay 6", "Relay 7", "Relay 8", "Relay 9", "Relay 10", "Relay 11", "Relay 12"]; "Relay Functions"."Remote"."Card Index" items=["Card 1", "Card 2", "Card 3", "Card 4", "Card 5"]; "Relay Functions"."Remote"."Relay Index" items=["Relay 1", "Relay 2", "Relay 3", "Relay 4", "Relay 5", "Relay 6", "Relay 7", "Relay 8", "Relay 9", "Relay 10", "Relay 11", "Relay 12"]}
  in  "P gas":T10={"Relay Functions"={"Remote"={"Card Index"=2, "Relay Index"=0}, "Active"={"Card Index"=2, "Relay Index"=1}, "Gas in"={"Card Index"=2, "Relay Index"=2}, "H2 flush"={"Card Index"=2, "Relay Index"=3}, "Run"={"Card Index"=2, "Relay Index"=4}}, "D/A Functions"={"Flow"={"Card Index"=1, "Channel Index"=2}}, "Flow Range"={"Flow (PGMFC1)"=1}, "A/D Functions"={"Flow"=5}} {"A/D Functions"."Flow" items=["Channel 1", "Channel 2", "Channel 3", "Channel 4", "Channel 5", "Channel 6", "Channel 7", "Channel 8", "Channel 9", "Channel 10", "Channel 11", "Channel 12", "Channel 13", "Channel 14", "Channel 15", "Channel 16"]; "Flow Range"."Flow (PGMFC1)" items=["0-10 sccm", "0-100 sccm", "0-1000 sccm"]; "D/A Functions"."Flow"."Card Index" items=["Card 1", "Card 2", "Card 3", "Card 4", "Card 5", "Card 6"]; "D/A Functions"."Flow"."Channel Index" items=["Channel 1", "Channel 2", "Channel 3", "Channel 4"]; "Relay Functions"."Run"."Card Index" items=["Card 1", "Card 2", "Card 3", "Card 4", "Card 5"]; "Relay Functions"."Run"."Relay Index" items=["Relay 1", "Relay 2", "Relay 3", "Relay 4", "Relay 5", "Relay 6", "Relay 7", "Relay 8", "Relay 9", "Relay 10", "Relay 11", "Relay 12"]; "Relay Functions"."H2 flush"."Card Index" items=["Card 1", "Card 2", "Card 3", "Card 4", "Card 5"]; "Relay Functions"."H2 flush"."Relay Index" items=["Relay 1", "Relay 2", "Relay 3", "Relay 4", "Relay 5", "Relay 6", "Relay 7", "Relay 8", "Relay 9", "Relay 10", "Relay 11", "Relay 12"]; "Relay Functions"."Gas in"."Card Index" items=["Card 1", "Card 2", "Card 3", "Card 4", "Card 5"]; "Relay Functions"."Gas in"."Relay Index" items=["Relay 1", "Relay 2", "Relay 3", "Relay 4", "Relay 5", "Relay 6", "Relay 7", "Relay 8", "Relay 9", "Relay 10", "Relay 11", "Relay 12"]; "Relay Functions"."Active"."Card Index" items=["Card 1", "Card 2", "Card 3", "Card 4", "Card 5"]; "Relay Functions"."Active"."Relay Index" items=["Relay 1", "Relay 2", "Relay 3", "Relay 4", "Relay 5", "Relay 6", "Relay 7", "Relay 8", "Relay 9", "Relay 10", "Relay 11", "Relay 12"]; "Relay Functions"."Remote"."Card Index" items=["Card 1", "Card 2", "Card 3", "Card 4", "Card 5"]; "Relay Functions"."Remote"."Relay Index" items=["Relay 1", "Relay 2", "Relay 3", "Relay 4", "Relay 5", "Relay 6", "Relay 7", "Relay 8", "Relay 9", "Relay 10", "Relay 11", "Relay 12"]}
  in  "As gas":T11={"Relay Functions"={"Remote"={"Card Index"=2, "Relay Index"=5}, "Active"={"Card Index"=2, "Relay Index"=6}, "Gas in"={"Card Index"=2, "Relay Index"=7}, "H2 flush"={"Card Index"=2, "Relay Index"=8}, "Run"={"Card Index"=2, "Relay Index"=9}}, "D/A Functions"={"Flow"={"Card Index"=4, "Channel Index"=3}}, "Flow Range"={"Flow (ASGMFC1)"=0}, "A/D Functions"={"Flow"=6}} {"A/D Functions"."Flow" items=["Channel 1", "Channel 2", "Channel 3", "Channel 4", "Channel 5", "Channel 6", "Channel 7", "Channel 8", "Channel 9", "Channel 10", "Channel 11", "Channel 12", "Channel 13", "Channel 14", "Channel 15", "Channel 16"]; "Flow Range"."Flow (ASGMFC1)" items=["0-10 sccm", "0-100 sccm", "0-1000 sccm"]; "D/A Functions"."Flow"."Card Index" items=["Card 1", "Card 2", "Card 3", "Card 4", "Card 5", "Card 6"]; "D/A Functions"."Flow"."Channel Index" items=["Channel 1", "Channel 2", "Channel 3", "Channel 4"]; "Relay Functions"."Run"."Card Index" items=["Card 1", "Card 2", "Card 3", "Card 4", "Card 5"]; "Relay Functions"."Run"."Relay Index" items=["Relay 1", "Relay 2", "Relay 3", "Relay 4", "Relay 5", "Relay 6", "Relay 7", "Relay 8", "Relay 9", "Relay 10", "Relay 11", "Relay 12"]; "Relay Functions"."H2 flush"."Card Index" items=["Card 1", "Card 2", "Card 3", "Card 4", "Card 5"]; "Relay Functions"."H2 flush"."Relay Index" items=["Relay 1", "Relay 2", "Relay 3", "Relay 4", "Relay 5", "Relay 6", "Relay 7", "Relay 8", "Relay 9", "Relay 10", "Relay 11", "Relay 12"]; "Relay Functions"."Gas in"."Card Index" items=["Card 1", "Card 2", "Card 3", "Card 4", "Card 5"]; "Relay Functions"."Gas in"."Relay Index" items=["Relay 1", "Relay 2", "Relay 3", "Relay 4", "Relay 5", "Relay 6", "Relay 7", "Relay 8", "Relay 9", "Relay 10", "Relay 11", "Relay 12"]; "Relay Functions"."Active"."Card Index" items=["Card 1", "Card 2", "Card 3", "Card 4", "Card 5"]; "Relay Functions"."Active"."Relay Index" items=["Relay 1", "Relay 2", "Relay 3", "Relay 4", "Relay 5", "Relay 6", "Relay 7", "Relay 8", "Relay 9", "Relay 10", "Relay 11", "Relay 12"]; "Relay Functions"."Remote"."Card Index" items=["Card 1", "Card 2", "Card 3", "Card 4", "Card 5"]; "Relay Functions"."Remote"."Relay Index" items=["Relay 1", "Relay 2", "Relay 3", "Relay 4", "Relay 5", "Relay 6", "Relay 7", "Relay 8", "Relay 9", "Relay 10", "Relay 11", "Relay 12"]}
  in  "P bubbler":T12={"Relay Functions"={"Remote"={"Card Index"=1, "Relay Index"=0}, "Active"={"Card Index"=1, "Relay Index"=1}, "Bubbler In"={"Card Index"=1, "Relay Index"=2}, "Run"={"Card Index"=1, "Relay Index"=3}}, "D/A Functions"={"Flow"={"Card Index"=1, "Channel Index"=0}}, "Flow Ranges"={"Flow (PLMFC1)"=1}, "A/D Functions"={"Flow"=3}} {"A/D Functions"."Flow" items=["Channel 1", "Channel 2", "Channel 3", "Channel 4", "Channel 5", "Channel 6", "Channel 7", "Channel 8", "Channel 9", "Channel 10", "Channel 11", "Channel 12", "Channel 13", "Channel 14", "Channel 15", "Channel 16"]; "Flow Ranges"."Flow (PLMFC1)" items=["0-10 sccm", "0-100 sccm", "0-1000 sccm"]; "D/A Functions"."Flow"."Card Index" items=["Card 1", "Card 2", "Card 3", "Card 4", "Card 5", "Card 6"]; "D/A Functions"."Flow"."Channel Index" items=["Channel 1", "Channel 2", "Channel 3", "Channel 4"]; "Relay Functions"."Run"."Card Index" items=["Card 1", "Card 2", "Card 3", "Card 4", "Card 5"]; "Relay Functions"."Run"."Relay Index" items=["Relay 1", "Relay 2", "Relay 3", "Relay 4", "Relay 5", "Relay 6", "Relay 7", "Relay 8", "Relay 9", "Relay 10", "Relay 11", "Relay 12"]; "Relay Functions"."Bubbler In"."Card Index" items=["Card 1", "Card 2", "Card 3", "Card 4", "Card 5"]; "Relay Functions"."Bubbler In"."Relay Index" items=["Relay 1", "Relay 2", "Relay 3", "Relay 4", "Relay 5", "Relay 6", "Relay 7", "Relay 8", "Relay 9", "Relay 10", "Relay 11", "Relay 12"]; "Relay Functions"."Active"."Card Index" items=["Card 1", "Card 2", "Card 3", "Card 4", "Card 5"]; "Relay Functions"."Active"."Relay Index" items=["Relay 1", "Relay 2", "Relay 3", "Relay 4", "Relay 5", "Relay 6", "Relay 7", "Relay 8", "Relay 9", "Relay 10", "Relay 11", "Relay 12"]; "Relay Functions"."Remote"."Card Index" items=["Card 1", "Card 2", "Card 3", "Card 4", "Card 5"]; "Relay Functions"."Remote"."Relay Index" items=["Relay 1", "Relay 2", "Relay 3", "Relay 4", "Relay 5", "Relay 6", "Relay 7", "Relay 8", "Relay 9", "Relay 10", "Relay 11", "Relay 12"]}
  in  "Plasma feed":T13={"Relay Functions"={"Remote"={"Card Index"=1, "Relay Index"=4}, "Active"={"Card Index"=1, "Relay Index"=5}, "Bubbler In"={"Card Index"=1, "Relay Index"=6}, "Run"={"Card Index"=1, "Relay Index"=7}}, "D/A Functions"={"Flow"={"Card Index"=1, "Channel Index"=1}}, "Flow Ranges"={"Flow (ASLMFC1)"=2}, "A/D Functions"={"Flow"=3}} {"A/D Functions"."Flow" items=["Channel 1", "Channel 2", "Channel 3", "Channel 4", "Channel 5", "Channel 6", "Channel 7", "Channel 8", "Channel 9", "Channel 10", "Channel 11", "Channel 12", "Channel 13", "Channel 14", "Channel 15", "Channel 16"]; "Flow Ranges"."Flow (ASLMFC1)" items=["0-10 sccm", "0-100 sccm", "0-1000 sccm"]; "D/A Functions"."Flow"."Card Index" items=["Card 1", "Card 2", "Card 3", "Card 4", "Card 5", "Card 6"]; "D/A Functions"."Flow"."Channel Index" items=["Channel 1", "Channel 2", "Channel 3", "Channel 4"]; "Relay Functions"."Run"."Card Index" items=["Card 1", "Card 2", "Card 3", "Card 4", "Card 5"]; "Relay Functions"."Run"."Relay Index" items=["Relay 1", "Relay 2", "Relay 3", "Relay 4", "Relay 5", "Relay 6", "Relay 7", "Relay 8", "Relay 9", "Relay 10", "Relay 11", "Relay 12"]; "Relay Functions"."Bubbler In"."Card Index" items=["Card 1", "Card 2", "Card 3", "Card 4", "Card 5"]; "Relay Functions"."Bubbler In"."Relay Index" items=["Relay 1", "Relay 2", "Relay 3", "Relay 4", "Relay 5", "Relay 6", "Relay 7", "Relay 8", "Relay 9", "Relay 10", "Relay 11", "Relay 12"]; "Relay Functions"."Active"."Card Index" items=["Card 1", "Card 2", "Card 3", "Card 4", "Card 5"]; "Relay Functions"."Active"."Relay Index" items=["Relay 1", "Relay 2", "Relay 3", "Relay 4", "Relay 5", "Relay 6", "Relay 7", "Relay 8", "Relay 9", "Relay 10", "Relay 11", "Relay 12"]; "Relay Functions"."Remote"."Card Index" items=["Card 1", "Card 2", "Card 3", "Card 4", "Card 5"]; "Relay Functions"."Remote"."Relay Index" items=["Relay 1", "Relay 2", "Relay 3", "Relay 4", "Relay 5", "Relay 6", "Relay 7", "Relay 8", "Relay 9", "Relay 10", "Relay 11", "Relay 12"]}
  in  "Fe":T14={"Relay Functions"={"Remote"={"Card Index"=3, "Relay Index"=0}, "Active"={"Card Index"=3, "Relay Index"=1}, "Bubbler In"={"Card Index"=3, "Relay Index"=2}, "H2 dilute"={"Card Index"=3, "Relay Index"=4}, "Run"={"Card Index"=3, "Relay Index"=3}}, "D/A Functions"={"Flow 1"={"Card Index"=0, "Channel Index"=2}, "Flow 2"={"Card Index"=4, "Channel Index"=1}, "Flow 3"={"Card Index"=4, "Channel Index"=2}}, "Flow Ranges"={"Flow 1 (FEMFC1)"=0, "Flow 2 (FEMFC2)"=1, "Flow 3 (FEMFC3)"=2}, "A/D Functions"={"Flow 1"=3, "Flow 2"=3, "Flow 3"=3}} {"A/D Functions"."Flow 3" items=["Channel 1", "Channel 2", "Channel 3", "Channel 4", "Channel 5", "Channel 6", "Channel 7", "Channel 8", "Channel 9", "Channel 10", "Channel 11", "Channel 12", "Channel 13", "Channel 14", "Channel 15", "Channel 16"]; "A/D Functions"."Flow 2" items=["Channel 1", "Channel 2", "Channel 3", "Channel 4", "Channel 5", "Channel 6", "Channel 7", "Channel 8", "Channel 9", "Channel 10", "Channel 11", "Channel 12", "Channel 13", "Channel 14", "Channel 15", "Channel 16"]; "A/D Functions"."Flow 1" items=["Channel 1", "Channel 2", "Channel 3", "Channel 4", "Channel 5", "Channel 6", "Channel 7", "Channel 8", "Channel 9", "Channel 10", "Channel 11", "Channel 12", "Channel 13", "Channel 14", "Channel 15", "Channel 16"]; "Flow Ranges"."Flow 3 (FEMFC3)" items=["0-10 sccm", "0-100 sccm", "0-1000 sccm"]; "Flow Ranges"."Flow 2 (FEMFC2)" items=["0-10 sccm", "0-100 sccm", "0-1000 sccm"]; "Flow Ranges"."Flow 1 (FEMFC1)" items=["0-10 sccm", "0-100 sccm", "0-1000 sccm"]; "D/A Functions"."Flow 3"."Card Index" items=["Card 1", "Card 2", "Card 3", "Card 4", "Card 5", "Card 6"]; "D/A Functions"."Flow 3"."Channel Index" items=["Channel 1", "Channel 2", "Channel 3", "Channel 4"]; "D/A Functions"."Flow 2"."Card Index" items=["Card 1", "Card 2", "Card 3", "Card 4", "Card 5", "Card 6"]; "D/A Functions"."Flow 2"."Channel Index" items=["Channel 1", "Channel 2", "Channel 3", "Channel 4"]; "D/A Functions"."Flow 1"."Card Index" items=["Card 1", "Card 2", "Card 3", "Card 4", "Card 5", "Card 6"]; "D/A Functions"."Flow 1"."Channel Index" items=["Channel 1", "Channel 2", "Channel 3", "Channel 4"]; "Relay Functions"."Run"."Card Index" items=["Card 1", "Card 2", "Card 3", "Card 4", "Card 5"]; "Relay Functions"."Run"."Relay Index" items=["Relay 1", "Relay 2", "Relay 3", "Relay 4", "Relay 5", "Relay 6", "Relay 7", "Relay 8", "Relay 9", "Relay 10", "Relay 11", "Relay 12"]; "Relay Functions"."H2 dilute"."Card Index" items=["Card 1", "Card 2", "Card 3", "Card 4", "Card 5"]; "Relay Functions"."H2 dilute"."Relay Index" items=["Relay 1", "Relay 2", "Relay 3", "Relay 4", "Relay 5", "Relay 6", "Relay 7", "Relay 8", "Relay 9", "Relay 10", "Relay 11", "Relay 12"]; "Relay Functions"."Bubbler In"."Card Index" items=["Card 1", "Card 2", "Card 3", "Card 4", "Card 5"]; "Relay Functions"."Bubbler In"."Relay Index" items=["Relay 1", "Relay 2", "Relay 3", "Relay 4", "Relay 5", "Relay 6", "Relay 7", "Relay 8", "Relay 9", "Relay 10", "Relay 11", "Relay 12"]; "Relay Functions"."Active"."Card Index" items=["Card 1", "Card 2", "Card 3", "Card 4", "Card 5"]; "Relay Functions"."Active"."Relay Index" items=["Relay 1", "Relay 2", "Relay 3", "Relay 4", "Relay 5", "Relay 6", "Relay 7", "Relay 8", "Relay 9", "Relay 10", "Relay 11", "Relay 12"]; "Relay Functions"."Remote"."Card Index" items=["Card 1", "Card 2", "Card 3", "Card 4", "Card 5"]; "Relay Functions"."Remote"."Relay Index" items=["Relay 1", "Relay 2", "Relay 3", "Relay 4", "Relay 5", "Relay 6", "Relay 7", "Relay 8", "Relay 9", "Relay 10", "Relay 11", "Relay 12"]}
  in  "dopants":enum32{"p dopant", "n dopant", "both"}(tab)
  in  "p dopant":T15={"Relay Functions"={"Remote"={"Card Index"=4, "Relay Index"=0}, "Active"={"Card Index"=4, "Relay Index"=1}, "Bubbler In"={"Card Index"=4, "Relay Index"=2}, "H2 dilute"={"Card Index"=4, "Relay Index"=4}, "Gas in"={"Card Index"=4, "Relay Index"=5}, "Run"={"Card Index"=4, "Relay Index"=3}}, "D/A Functions"={"Flow 1"={"Card Index"=3, "Channel Index"=1}, "Flow 2"={"Card Index"=3, "Channel Index"=2}, "Flow 3"={"Card Index"=3, "Channel Index"=3}}, "Flow Ranges"={"Flow 1 (PDOPMFC1)"=1, "Flow 2 (PDOPMFC2)"=1, "Flow 3 (PDOPMFC3)"=2, "Gas flow (PDOPMFC4)"=1}} {"Flow Ranges"."Gas flow (PDOPMFC4)" items=["0-10 sccm", "0-100 sccm", "0-1000 sccm"]; "Flow Ranges"."Flow 3 (PDOPMFC3)" items=["0-10 sccm", "0-100 sccm", "0-1000 sccm"]; "Flow Ranges"."Flow 2 (PDOPMFC2)" items=["0-10 sccm", "0-100 sccm", "0-1000 sccm"]; "Flow Ranges"."Flow 1 (PDOPMFC1)" items=["0-10 sccm", "0-100 sccm", "0-1000 sccm"]; "D/A Functions"."Flow 3"."Card Index" items=["Card 1", "Card 2", "Card 3", "Card 4", "Card 5", "Card 6"]; "D/A Functions"."Flow 3"."Channel Index" items=["Channel 1", "Channel 2", "Channel 3", "Channel 4"]; "D/A Functions"."Flow 2"."Card Index" items=["Card 1", "Card 2", "Card 3", "Card 4", "Card 5", "Card 6"]; "D/A Functions"."Flow 2"."Channel Index" items=["Channel 1", "Channel 2", "Channel 3", "Channel 4"]; "D/A Functions"."Flow 1"."Card Index" items=["Card 1", "Card 2", "Card 3", "Card 4", "Card 5", "Card 6"]; "D/A Functions"."Flow 1"."Channel Index" items=["Channel 1", "Channel 2", "Channel 3", "Channel 4"]; "Relay Functions"."Run"."Card Index" items=["Card 1", "Card 2", "Card 3", "Card 4", "Card 5"]; "Relay Functions"."Run"."Relay Index" items=["Relay 1", "Relay 2", "Relay 3", "Relay 4", "Relay 5", "Relay 6", "Relay 7", "Relay 8", "Relay 9", "Relay 10", "Relay 11", "Relay 12"]; "Relay Functions"."Gas in"."Card Index" items=["Card 1", "Card 2", "Card 3", "Card 4", "Card 5"]; "Relay Functions"."Gas in"."Relay Index" items=["Relay 1", "Relay 2", "Relay 3", "Relay 4", "Relay 5", "Relay 6", "Relay 7", "Relay 8", "Relay 9", "Relay 10", "Relay 11", "Relay 12"]; "Relay Functions"."H2 dilute"."Card Index" items=["Card 1", "Card 2", "Card 3", "Card 4", "Card 5"]; "Relay Functions"."H2 dilute"."Relay Index" items=["Relay 1", "Relay 2", "Relay 3", "Relay 4", "Relay 5", "Relay 6", "Relay 7", "Relay 8", "Relay 9", "Relay 10", "Relay 11", "Relay 12"]; "Relay Functions"."Bubbler In"."Card Index" items=["Card 1", "Card 2", "Card 3", "Card 4", "Card 5"]; "Relay Functions"."Bubbler In"."Relay Index" items=["Relay 1", "Relay 2", "Relay 3", "Relay 4", "Relay 5", "Relay 6", "Relay 7", "Relay 8", "Relay 9", "Relay 10", "Relay 11", "Relay 12"]; "Relay Functions"."Active"."Card Index" items=["Card 1", "Card 2", "Card 3", "Card 4", "Card 5"]; "Relay Functions"."Active"."Relay Index" items=["Relay 1", "Relay 2", "Relay 3", "Relay 4", "Relay 5", "Relay 6", "Relay 7", "Relay 8", "Relay 9", "Relay 10", "Relay 11", "Relay 12"]; "Relay Functions"."Remote"."Card Index" items=["Card 1", "Card 2", "Card 3", "Card 4", "Card 5"]; "Relay Functions"."Remote"."Relay Index" items=["Relay 1", "Relay 2", "Relay 3", "Relay 4", "Relay 5", "Relay 6", "Relay 7", "Relay 8", "Relay 9", "Relay 10", "Relay 11", "Relay 12"]}
  in  "n dopant":T16={"Relay Functions"={"Remote"={"Card Index"=4, "Relay Index"=6}, "Active"={"Card Index"=4, "Relay Index"=7}, "Bubbler In"={"Card Index"=4, "Relay Index"=8}, "H2 dilute"={"Card Index"=4, "Relay Index"=10}, "Gas in"={"Card Index"=4, "Relay Index"=11}, "Run 2"={"Card Index"=4, "Relay Index"=10}}, "D/A Functions"={"Flow 1"={"Card Index"=2, "Channel Index"=2}, "Flow 2"={"Card Index"=1, "Channel Index"=3}, "Flow 3"={"Card Index"=3, "Channel Index"=0}}, "Flow Ranges"={"Flow 1 (NDOPMFC1)"=1, "Flow 2 (NDOPMFC2)"=1, "Flow 3 (NDOPMFC3)"=2, "Gas flow (NDOPMFC4)"=1}} {"Flow Ranges"."Gas flow (NDOPMFC4)" items=["0-10 sccm", "0-100 sccm", "0-1000 sccm"]; "Flow Ranges"."Flow 3 (NDOPMFC3)" items=["0-10 sccm", "0-100 sccm", "0-1000 sccm"]; "Flow Ranges"."Flow 2 (NDOPMFC2)" items=["0-10 sccm", "0-100 sccm", "0-1000 sccm"]; "Flow Ranges"."Flow 1 (NDOPMFC1)" items=["0-10 sccm", "0-100 sccm", "0-1000 sccm"]; "D/A Functions"."Flow 3"."Card Index" items=["Card 1", "Card 2", "Card 3", "Card 4", "Card 5", "Card 6"]; "D/A Functions"."Flow 3"."Channel Index" items=["Channel 1", "Channel 2", "Channel 3", "Channel 4"]; "D/A Functions"."Flow 2"."Card Index" items=["Card 1", "Card 2", "Card 3", "Card 4", "Card 5", "Card 6"]; "D/A Functions"."Flow 2"."Channel Index" items=["Channel 1", "Channel 2", "Channel 3", "Channel 4"]; "D/A Functions"."Flow 1"."Card Index" items=["Card 1", "Card 2", "Card 3", "Card 4", "Card 5", "Card 6"]; "D/A Functions"."Flow 1"."Channel Index" items=["Channel 1", "Channel 2", "Channel 3", "Channel 4"]; "Relay Functions"."Run 2"."Card Index" items=["Card 1", "Card 2", "Card 3", "Card 4", "Card 5"]; "Relay Functions"."Run 2"."Relay Index" items=["Relay 1", "Relay 2", "Relay 3", "Relay 4", "Relay 5", "Relay 6", "Relay 7", "Relay 8", "Relay 9", "Relay 10", "Relay 11", "Relay 12"]; "Relay Functions"."Gas in"."Card Index" items=["Card 1", "Card 2", "Card 3", "Card 4", "Card 5"]; "Relay Functions"."Gas in"."Relay Index" items=["Relay 1", "Relay 2", "Relay 3", "Relay 4", "Relay 5", "Relay 6", "Relay 7", "Relay 8", "Relay 9", "Relay 10", "Relay 11", "Relay 12"]; "Relay Functions"."H2 dilute"."Card Index" items=["Card 1", "Card 2", "Card 3", "Card 4", "Card 5"]; "Relay Functions"."H2 dilute"."Relay Index" items=["Relay 1", "Relay 2", "Relay 3", "Relay 4", "Relay 5", "Relay 6", "Relay 7", "Relay 8", "Relay 9", "Relay 10", "Relay 11", "Relay 12"]; "Relay Functions"."Bubbler In"."Card Index" items=["Card 1", "Card 2", "Card 3", "Card 4", "Card 5"]; "Relay Functions"."Bubbler In"."Relay Index" items=["Relay 1", "Relay 2", "Relay 3", "Relay 4", "Relay 5", "Relay 6", "Relay 7", "Relay 8", "Relay 9", "Relay 10", "Relay 11", "Relay 12"]; "Relay Functions"."Active"."Card Index" items=["Card 1", "Card 2", "Card 3", "Card 4", "Card 5"]; "Relay Functions"."Active"."Relay Index" items=["Relay 1", "Relay 2", "Relay 3", "Relay 4", "Relay 5", "Relay 6", "Relay 7", "Relay 8", "Relay 9", "Relay 10", "Relay 11", "Relay 12"]; "Relay Functions"."Remote"."Card Index" items=["Card 1", "Card 2", "Card 3", "Card 4", "Card 5"]; "Relay Functions"."Remote"."Relay Index" items=["Relay 1", "Relay 2", "Relay 3", "Relay 4", "Relay 5", "Relay 6", "Relay 7", "Relay 8", "Relay 9", "Relay 10", "Relay 11", "Relay 12"]}
  in  "p/n dopants":T17={"Relay Functions"={"Output"={"Card Index"=3, "Relay Index"=10}}, "A/D Functions"={"Flow 1"=13, "Flow 2"=14, "Flow 3"=15}} {"A/D Functions"."Flow 3" items=["Channel 1", "Channel 2", "Channel 3", "Channel 4", "Channel 5", "Channel 6", "Channel 7", "Channel 8", "Channel 9", "Channel 10", "Channel 11", "Channel 12", "Channel 13", "Channel 14", "Channel 15", "Channel 16"]; "A/D Functions"."Flow 2" items=["Channel 1", "Channel 2", "Channel 3", "Channel 4", "Channel 5", "Channel 6", "Channel 7", "Channel 8", "Channel 9", "Channel 10", "Channel 11", "Channel 12", "Channel 13", "Channel 14", "Channel 15", "Channel 16"]; "A/D Functions"."Flow 1" items=["Channel 1", "Channel 2", "Channel 3", "Channel 4", "Channel 5", "Channel 6", "Channel 7", "Channel 8", "Channel 9", "Channel 10", "Channel 11", "Channel 12", "Channel 13", "Channel 14", "Channel 15", "Channel 16"]; "Relay Functions"."Output"."Card Index" items=["Card 1", "Card 2", "Card 3", "Card 4", "Card 5"]; "Relay Functions"."Output"."Relay Index" items=["Relay 1", "Relay 2", "Relay 3", "Relay 4", "Relay 5", "Relay 6", "Relay 7", "Relay 8", "Relay 9", "Relay 10", "Relay 11", "Relay 12"]}
  in  "Vacuum":T18={"Relay Functions"={"Remote"={"Card Index"=1, "Relay Index"=8}, "Atm"={"Card Index"=1, "Relay Index"=9}, "Exhaust"={"Card Index"=1, "Relay Index"=10}}} {"Relay Functions"."Exhaust"."Card Index" items=["Card 1", "Card 2", "Card 3", "Card 4", "Card 5"]; "Relay Functions"."Exhaust"."Relay Index" items=["Relay 1", "Relay 2", "Relay 3", "Relay 4", "Relay 5", "Relay 6", "Relay 7", "Relay 8", "Relay 9", "Relay 10", "Relay 11", "Relay 12"]; "Relay Functions"."Atm"."Card Index" items=["Card 1", "Card 2", "Card 3", "Card 4", "Card 5"]; "Relay Functions"."Atm"."Relay Index" items=["Relay 1", "Relay 2", "Relay 3", "Relay 4", "Relay 5", "Relay 6", "Relay 7", "Relay 8", "Relay 9", "Relay 10", "Relay 11", "Relay 12"]; "Relay Functions"."Remote"."Card Index" items=["Card 1", "Card 2", "Card 3", "Card 4", "Card 5"]; "Relay Functions"."Remote"."Relay Index" items=["Relay 1", "Relay 2", "Relay 3", "Relay 4", "Relay 5", "Relay 6", "Relay 7", "Relay 8", "Relay 9", "Relay 10", "Relay 11", "Relay 12"]}
  in  "Heater/Spinner":T19={"Relay Functions"={"Remote"={"Card Index"=1, "Relay Index"=8}, "Heater on"={"Card Index"=1, "Relay Index"=9}, "Spinner on"={"Card Index"=1, "Relay Index"=10}}} {"Relay Functions"."Spinner on"."Card Index" items=["Card 1", "Card 2", "Card 3", "Card 4", "Card 5"]; "Relay Functions"."Spinner on"."Relay Index" items=["Relay 1", "Relay 2", "Relay 3", "Relay 4", "Relay 5", "Relay 6", "Relay 7", "Relay 8", "Relay 9", "Relay 10", "Relay 11", "Relay 12"]; "Relay Functions"."Heater on"."Card Index" items=["Card 1", "Card 2", "Card 3", "Card 4", "Card 5"]; "Relay Functions"."Heater on"."Relay Index" items=["Relay 1", "Relay 2", "Relay 3", "Relay 4", "Relay 5", "Relay 6", "Relay 7", "Relay 8", "Relay 9", "Relay 10", "Relay 11", "Relay 12"]; "Relay Functions"."Remote"."Card Index" items=["Card 1", "Card 2", "Card 3", "Card 4", "Card 5"]; "Relay Functions"."Remote"."Relay Index" items=["Relay 1", "Relay 2", "Relay 3", "Relay 4", "Relay 5", "Relay 6", "Relay 7", "Relay 8", "Relay 9", "Relay 10", "Relay 11", "Relay 12"]}
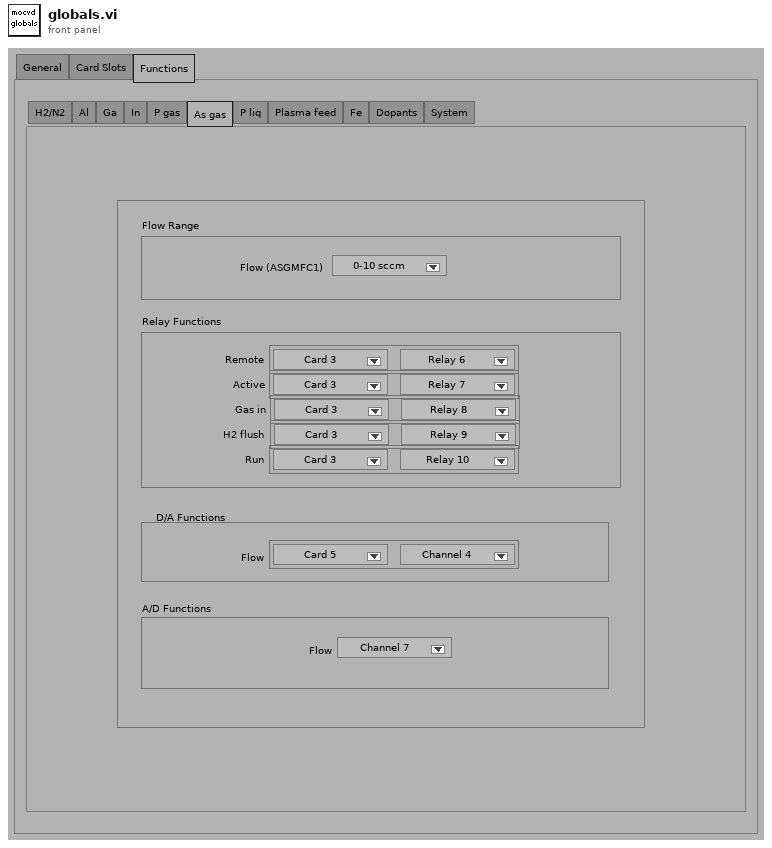
[diagram p1: front panel]
types:
  T1 = cluster{"Relay Card Slots":cluster{"Card 1":u16, "Card 2":u16, "Card 3":u16, "Card 4":u16, "Card 5":u16}, "A/D Card Slots":cluster{"Scanner":u16, "High-Speed A/D":u16, "Timer":u16}, "D/A Cards":cluster{"Quad (10-bit) D/A Card Slots":cluster{"Card 1":u16, "Card 2":u16, "Card 3":u16, "Card 4":u16, "Card 5":u16}, "Single (12-bit) D/A Card Slot":cluster{"Card 6":u16}}}
  T2 = enum32{"H2/N2", "Al", "Ga", "In", "P gas", "As gas", "P liq", "Plasma feed", "Fe", "Dopants", "System"}
  T3 = typedef "relaySpec.ctl" = cluster{"Card Index":u16, "Relay Index":u16}
  T4 = typedef "DA_Spec.ctl" = cluster{"Card Index":u16, "Channel Index":u16}
  T5 = typedef "AD_Spec.ctl" = u16
  T6 = cluster{"Relay Functions":cluster{"Remote":T3, "H2 active":T3, "N2 active":T3, "Output":T3}, "D/A Functions":cluster{"H2 flow":T4, "N2 flow":T4}, "Flow Ranges":cluster{"H2 flow (HMFC1)":u16, "N2 flow (NMFC1)":u16}, "A/D Functions":cluster{"H2/N2 flow":T5}}
  T7 = cluster{"Relay Functions":cluster{"Remote":T3, "Active":T3, "Bubbler In":T3, "Run":T3}, "D/A Functions":cluster{"Flow":T4}, "Flow Ranges":cluster{"Flow (AlMFC1)":u16}, "A/D Functions":cluster{"Flow":T5}}
  T8 = cluster{"Relay Functions":cluster{"Remote":T3, "Active":T3, "Bubbler In":T3, "H2 dilute":T3, "Run":T3}, "D/A Functions":cluster{"Flow 1":T4, "Flow 2":T4, "Flow 3":T4}, "Flow Ranges":cluster{"Flow 1 (GAMFC1)":u16, "Flow 2 (GAMFC2)":u16, "Flow 3 (GAMFC3)":u16}, "A/D Functions":cluster{"Flow 1":T5, "Flow 2":T5, "Flow 3":T5}}
  T9 = cluster{"Relay Functions":cluster{"Remote":T3, "Active":T3, "Bubbler In":T3, "Run":T3}, "D/A Functions":cluster{"Flow":T4}, "Flow Ranges":cluster{"Flow (INMFC1)":u16}, "A/D Functions":cluster{"Flow":T5}}
  T10 = cluster{"Relay Functions":cluster{"Remote":T3, "Active":T3, "Gas in":T3, "H2 flush":T3, "Run":T3}, "D/A Functions":cluster{"Flow":T4}, "Flow Range":cluster{"Flow (PGMFC1)":u16}, "A/D Functions":cluster{"Flow":T5}}
  T11 = cluster{"Relay Functions":cluster{"Remote":T3, "Active":T3, "Gas in":T3, "H2 flush":T3, "Run":T3}, "D/A Functions":cluster{"Flow":T4}, "Flow Range":cluster{"Flow (ASGMFC1)":u16}, "A/D Functions":cluster{"Flow":T5}}
  T12 = cluster{"Relay Functions":cluster{"Remote":T3, "Active":T3, "Bubbler In":T3, "Run":T3}, "D/A Functions":cluster{"Flow":T4}, "Flow Ranges":cluster{"Flow (PLMFC1)":u16}, "A/D Functions":cluster{"Flow":T5}}
  T13 = cluster{"Relay Functions":cluster{"Remote":T3, "Active":T3, "Bubbler In":T3, "Run":T3}, "D/A Functions":cluster{"Flow":T4}, "Flow Ranges":cluster{"Flow (ASLMFC1)":u16}, "A/D Functions":cluster{"Flow":T5}}
  T14 = cluster{"Relay Functions":cluster{"Remote":T3, "Active":T3, "Bubbler In":T3, "H2 dilute":T3, "Run":T3}, "D/A Functions":cluster{"Flow 1":T4, "Flow 2":T4, "Flow 3":T4}, "Flow Ranges":cluster{"Flow 1 (FEMFC1)":u16, "Flow 2 (FEMFC2)":u16, "Flow 3 (FEMFC3)":u16}, "A/D Functions":cluster{"Flow 1":T5, "Flow 2":T5, "Flow 3":T5}}
  T15 = cluster{"Relay Functions":cluster{"Remote":T3, "Active":T3, "Bubbler In":T3, "H2 dilute":T3, "Gas in":T3, "Run":T3}, "D/A Functions":cluster{"Flow 1":T4, "Flow 2":T4, "Flow 3":T4}, "Flow Ranges":cluster{"Flow 1 (PDOPMFC1)":u16, "Flow 2 (PDOPMFC2)":u16, "Flow 3 (PDOPMFC3)":u16, "Gas flow (PDOPMFC4)":u16}}
  T16 = cluster{"Relay Functions":cluster{"Remote":T3, "Active":T3, "Bubbler In":T3, "H2 dilute":T3, "Gas in":T3, "Run 2":T3}, "D/A Functions":cluster{"Flow 1":T4, "Flow 2":T4, "Flow 3":T4}, "Flow Ranges":cluster{"Flow 1 (NDOPMFC1)":u16, "Flow 2 (NDOPMFC2)":u16, "Flow 3 (NDOPMFC3)":u16, "Gas flow (NDOPMFC4)":u16}}
  T17 = cluster{"Relay Functions":cluster{"Output":T3}, "A/D Functions":cluster{"Flow 1":T5, "Flow 2":T5, "Flow 3":T5}}
  T18 = cluster{"Relay Functions":cluster{"Remote":T3, "Atm":T3, "Exhaust":T3}}
  T19 = cluster{"Relay Functions":cluster{"Remote":T3, "Heater on":T3, "Spinner on":T3}}
diagram:
